vi "bin single channel using bin col.vi"(0 "device data Spreadsheet format":string[][](array[string]), 1 "bin values":string[](array[string]), 2 "col name":string="Bin #") -> (3 "unique bin vals":string[](array[string]), 4 "bin vals wout blank data":string[](array[string]), 5 "Means":dbl[](array[numeric]), 6 "Sds":dbl[](array[numeric]))   [LabVIEW 2013]
uses:
  <userlib>/_OpenG.lib/array/array.llb/Search 1D Array (String)__ogtk.vi
  <userlib>/_OpenG.lib/array/array.llb/Delete Elements from 1D Array (String)__ogtk.vi
  <userlib>/_OpenG.lib/array/array.llb/Remove Duplicates from 1D Array (String)__ogtk.vi
  <userlib>/_OpenG.lib/array/array.llb/Delete Elements from 1D Array (DBL)__ogtk.vi
  <vilib>/Analysis/NI_AALBase.lvlib
panel:
  out "deleted elements":dbl[][](array[numeric])
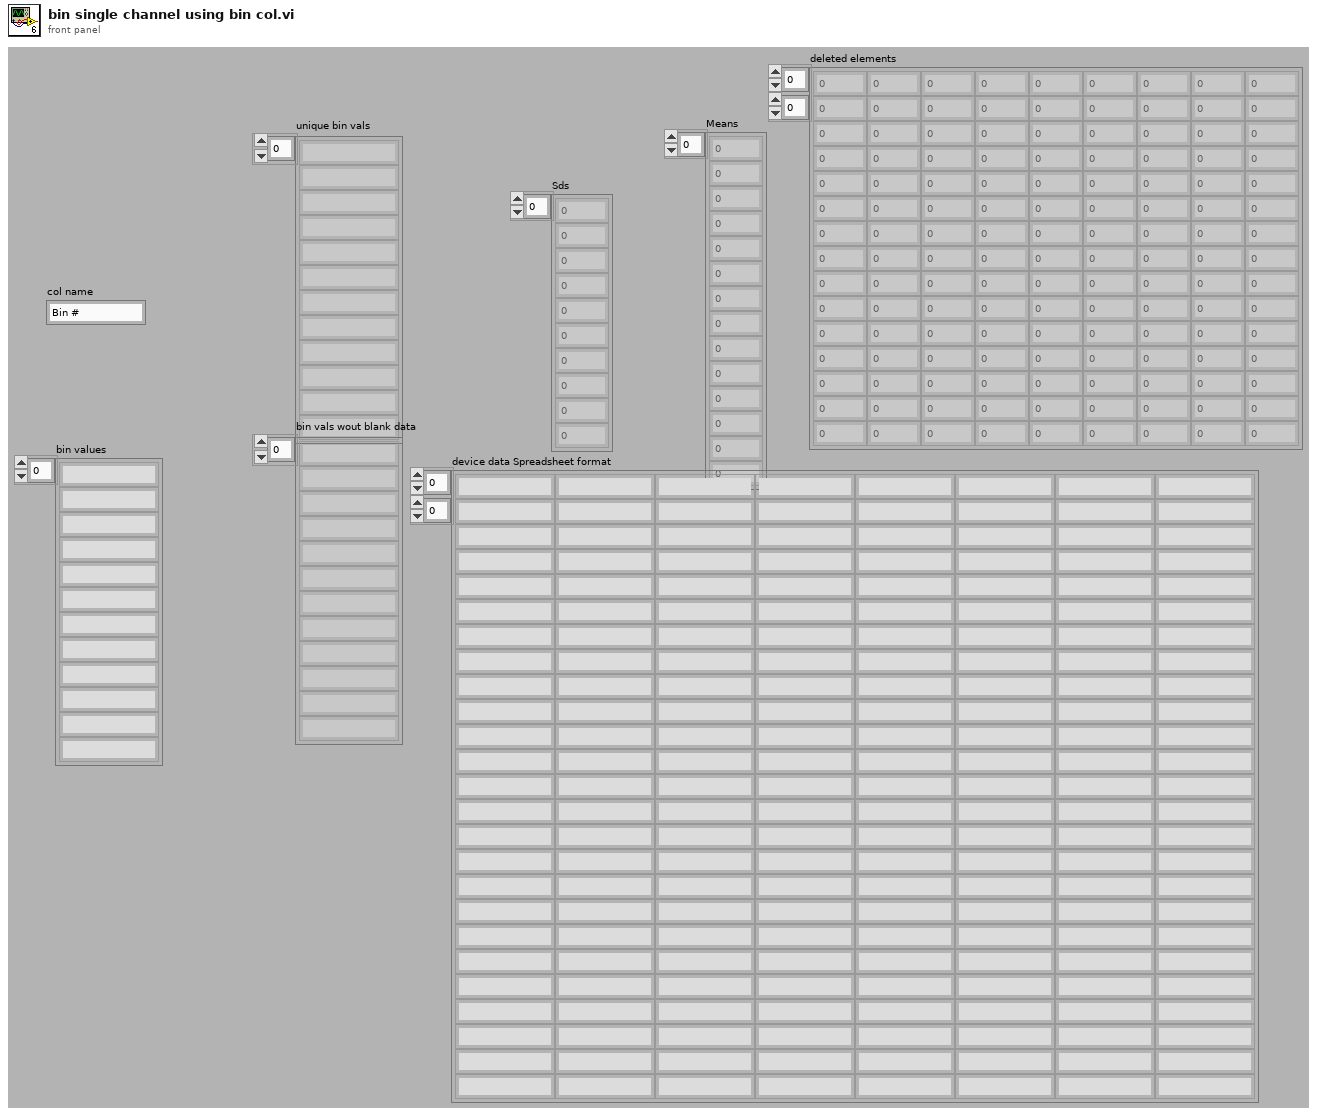
[diagram p1: front panel]
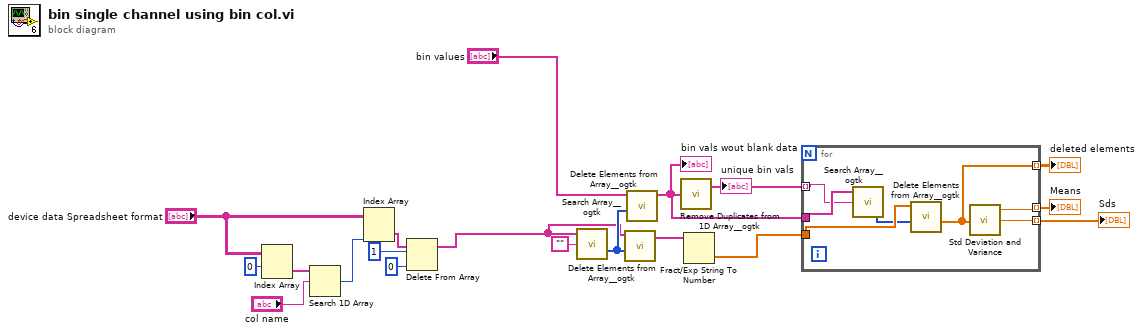
[diagram p0: block diagram]
diagram:
  n1 = Index Array(array="device data Spreadsheet format", index (row)=0) -> (element=w10:string[])  [unwired: 1 in]
  n2 = Search 1D Array(1D array=w10, element="col name") -> (index of element=w6:i32)  [unwired: 1 in]
  n3 = Index Array(array="device data Spreadsheet format", index (col)=w6) -> (element=w5:string[])  [unwired: 1 in]
  n4 = Delete From Array(array=w5, length=1, index=0) -> (array with subset deleted=w2:string[])  [unwired: 1 out]
  n5 = call-poly <userlib>:"Search Array__ogtk.vi"("Array"=w2, "Element Data"="") -> ("Indices of Elements"=w13:i32[])  [unwired: 7 in]
  n6 = call-poly <userlib>:"Delete Elements from Array__ogtk.vi"("indices"=w13, "array"=w2) -> ("array w/ subset deleted"=w16:string[])  [unwired: 8 in, 1 out]
  n7 = call-poly <userlib>:"Delete Elements from Array__ogtk.vi"("indices"=w13, "array"="bin values") -> ("array w/ subset deleted"=w15:string[])  [unwired: 8 in, 1 out]
  "bin vals wout blank data" <- w15
  n8 = call-poly <userlib>:"Remove Duplicates from 1D Array__ogtk.vi"("Input Array"=w15) -> ("Output Array"=w14:string[])  [unwired: 1 out]
  "unique bin vals" <- w14
  n9 = Fract/Exp String To Number(string=w16) -> (number=w17:dbl[])  [unwired: 3 in, 1 out]
  n10 = for {
    tunnel: w14 -> [w25] mode=indexing
    tunnel: w17 -> [w24]
    tunnel: w15 -> [w26]
    tunnel: [w22] -> w18 mode=indexing
    tunnel: [w21] -> w19 mode=indexing
    tunnel: [w20] -> w1 mode=indexing
    n11 = call-poly <userlib>:"Search Array__ogtk.vi"("Array"=w26, "Element Data"=w25) -> ("Indices of Elements"=w23:i32[])  [unwired: 7 in]
    n12 = call-poly <userlib>:"Delete Elements from Array__ogtk.vi"("indices"=w23, "array"=w24) -> ("deleted elements"=w20:dbl[])  [unwired: 8 in, 1 out]
    n13 = call <vilib>:"Std Deviation and Variance.vi"("X"=w20) -> ("mean"=w22:dbl, "standard deviation"=w21:dbl)  [unwired: 1 in, 1 out]
  }
  "Sds" <- w19
  "Means" <- w18
  "deleted elements" <- w1
